vi "Write Sub Panel Product.vi"(8 "error in (no error)":errorcluster, 10 "Sub Panel Product":refnum<vi>, 11 "Soda_Actor in":refnum<class "Soda_Actor.lvclass">) -> (0 "error out":errorcluster, 3 "Soda_Actor out":refnum<class "Soda_Actor.lvclass">)   [LabVIEW 2019, in "Soda_Actor.lvlib" / "Soda_Actor.lvclass"]
uses:
  Soda_Actor.lvclass
  Soda_Actor.lvclass/Soda_Actor.ctl
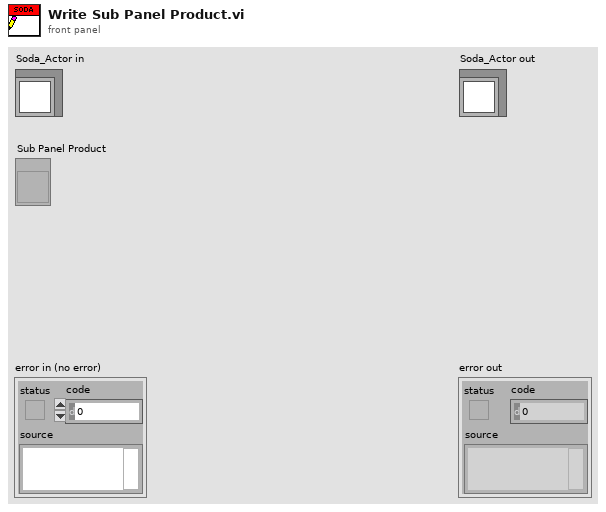
[diagram p1: front panel]
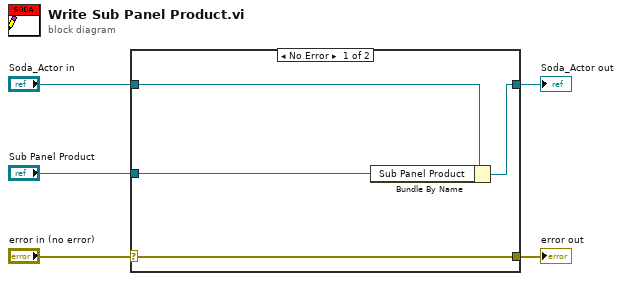
[diagram p0: block diagram]
diagram:
  n1 = case shown="No Error" "error in (no error)" {
    selector: "error in (no error)" -> [w9 w10]
    tunnel: [w9 w10] -> w4
    tunnel: [w7 w11] -> w2
    tunnel: "Soda_Actor in" -> [w8 w11]
    tunnel: "Sub Panel Product" -> [w6 _]
    frame No Error {
      n2 = Bundle By Name(cluster=w8, "Sub Panel Product"=w6) -> (w7:refnum<class "Soda_Actor.lvclass">)
    }
    frame Error {
    }
  }
  "error out" <- w4
  "Soda_Actor out" <- w2
